vi "Set Logical Channel Name and Color.vi"(6 "Logical Channel Color":u32(colorbox)=6618880, 8 "error in (no error)":errorcluster, 9 "Logical Channel Name":string, 10 "Logical Channel":u16(ring) items=["VL1", "VL2", "VL3", "VL4", "VL5", "VL6", "VL7", "VL8", "VL9", "VL10", "VL11", "VL12"], 11 "VISA resource name":refnum<visa-resource-name>) -> (0 "error out":errorcluster, 3 "VISA resource name out":refnum<visa-resource-name>)   [LabVIEW 2017, in "Sefram DAS220.lvlib"]
doc: "Change logical channel name and color.\nLogical channels (from VL1 to VL12) : <B>0 to 11</B>"
uses:
  <instrlib>/Sefram DAS220/Sefram DAS220.lvlib
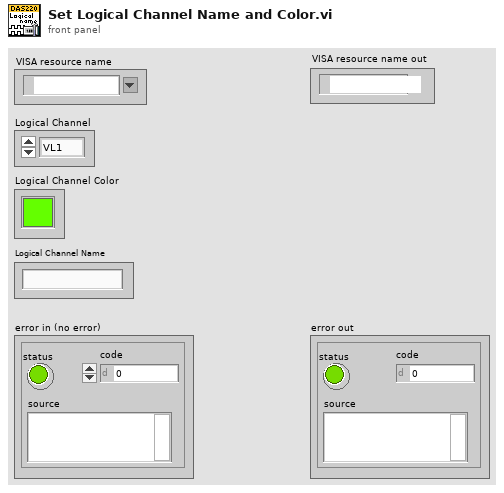
[diagram p1: front panel]
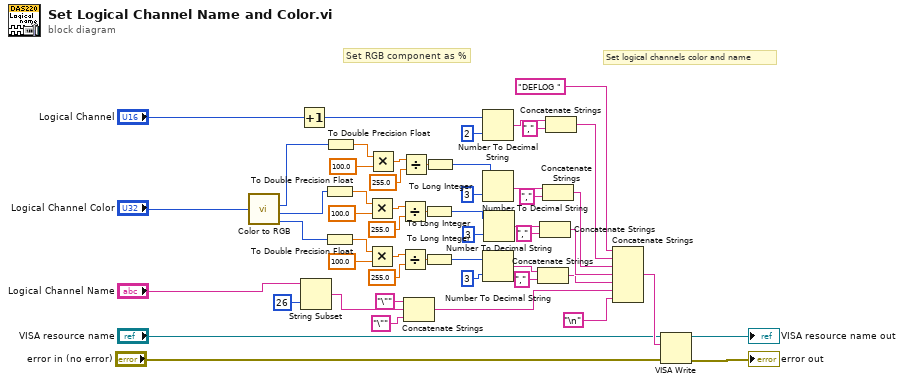
[diagram p0: block diagram]
diagram:
  # "Set RGB component as %"
  # "Set logical channels color and name"
  n1 = call <vilib>:"Color to RGB.vi"("Color"="Logical Channel Color") -> ("R"=w27:u8, "G"=w33:u8, "B"=w42:u8)  [unwired: 1 out]
  n2 = Increment(x="Logical Channel") -> (x+1=w22:u16)
  n3 = String Subset(string="Logical Channel Name", length (rest)=26 ("length (rest)")) -> (substring=w6:string)  [unwired: 1 in]
  n4 = To Double Precision Float(number=w33) -> (double precision float=w35:dbl)
  n5 = To Double Precision Float(number=w42) -> (double precision float=w41:dbl)
  n6 = To Double Precision Float(number=w27) -> (double precision float=w29:dbl)
  n7 = Multiply(x=w35, y=100.0) -> (x*y=w37:dbl)
  n8 = Multiply(x=w41, y=100.0) -> (x*y=w44:dbl)
  n9 = Multiply(x=w29, y=100.0) -> (x*y=w31:dbl)
  n10 = Divide(x=w37, y=255.0) -> (x/y=w34:dbl)
  n11 = Divide(x=w44, y=255.0) -> (x/y=w40:dbl)
  n12 = Divide(x=w31, y=255.0) -> (x/y=w28:dbl)
  n13 = Concatenate Strings("\"" ("string"), w6, "\"" ("string")) -> (w2:string)
  n14 = To Long Integer(number=w34) -> (32bit integer=w25:i32)
  n15 = To Long Integer(number=w40) -> (32bit integer=w39:i32)
  n16 = To Long Integer(number=w28) -> (32bit integer=w26:i32)
  n17 = Number To Decimal String(number=w22, width (-)=i16 2) -> (decimal integer string=w19:string)
  n18 = Number To Decimal String(number=w26, width (-)=i16 3) -> (decimal integer string=w15:string)
  n19 = Number To Decimal String(number=w39, width (-)=i16 3) -> (decimal integer string=w9:string)
  n20 = Number To Decimal String(number=w25, width (-)=i16 3) -> (decimal integer string=w12:string)
  n21 = Concatenate Strings(w9, "," ("string")) -> (w8:string)
  n22 = Concatenate Strings(w12, "," ("string")) -> (w11:string)
  n23 = Concatenate Strings(w15, "," ("string")) -> (w14:string)
  n24 = Concatenate Strings(w19, "," ("string")) -> (w18:string)
  n25 = Concatenate Strings("DEFLOG " ("string"), w18, w14, w11, w8, w2, "\n") -> (w53:string)
  n26 = VISA Write(VISA resource name="VISA resource name", write buffer=w53, error in (no error)="error in (no error)") -> (VISA resource name out=→"VISA resource name out":refnum<visa-resource-name>, error out=→"error out":errorcluster)  [unwired: 1 out]
